vi "NicmosMasks.vi"(2 "MASKBANKS":T1, 9 "Error in (no error)":errorcluster caption="error in (no error)") -> (6 "Error out":errorcluster caption="error out")   [LabVIEW 2009]
uses:
  Controls/NICMOS.MASKBANKS.ctl
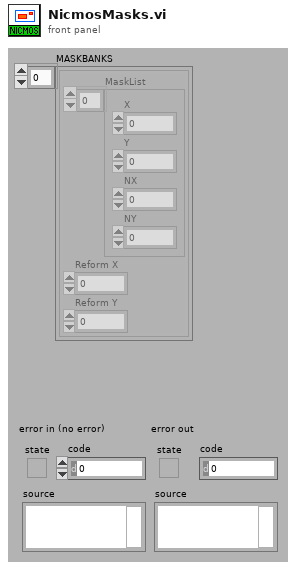
[diagram p1: front panel]
types:
  T1 = typedef "NICMOS.MASKBANKS.ctl" = cluster{"MaskList":cluster{"X":i32, "Y":i32, "NX":i32, "NY":i32}[], "Reform X":i32, "Reform Y":i32}[]
  T2 = cluster{"MaskList":cluster{"X":i32, "Y":i32, "NX":i32, "NY":i32}[], "Reform X":i32, "Reform Y":i32}
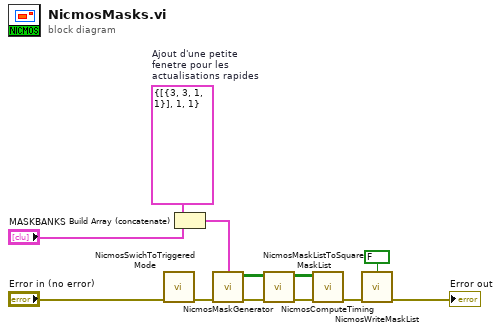
[diagram p0: block diagram]
diagram:
  w4 = T2 {"MaskList"=[{"X"=3, "Y"=3, "NX"=1, "NY"=1}], "Reform X"=1, "Reform Y"=1}  # Ajout d'une petite fenetre pour les actualisations rapides
  n1 = call "NicmosSwichToTriggeredMode.vi"("error in (no error)"="Error in (no error)") -> ("error out"=w10:errorcluster)  [unwired: 8 in]
  n2 = Build Array (concatenate)(w4, "MASKBANKS") -> (w2:T1)
  n3 = call "NicmosMaskGenerator.vi"("MASKBANKS"=w2, "error in (no error)"=w10) -> ("Mask List"=w3:bool[][][], "error out"=w11:errorcluster)  [unwired: 6 in]
  n4 = call "NicmosMaskListToSquareMaskList.vi"("Mask In [8x128x128]"=w3, "error in (no error)"=w11) -> ("Mask Out [8x128x128]"=w8:bool[][][], "error out"=w7:errorcluster)  [unwired: 6 in]
  n5 = call "NicmosComputeTiming.vi"("Mask In [8x128x128]"=w8, "error in"=w7) -> ("error out"=w9:errorcluster)  [unwired: 7 in]
  n6 = call "NicmosWriteMaskList.vi"("Force Write Mask"=FALSE, "error in"=w9) -> ("error out"=→"Error out":errorcluster)  [unwired: 7 in]
